vi "LinearSystemLoop_DCMotor_Execute.vi"(5 "LinearSystem_ID_DCMotor_Model":T2={"DCMOTOR_TYPES"=enum."NEO", "Num Motors"=1, "Gearing"=1.0, "MOI kgm2"=0.001} {"MOI kgm2" format="%#_13g"; "Gearing" format="%#_13g"}, 6 "dT Sec":dbl=0.02, 7 "LinearSystem_DCMotor_Ctrl_Params":T1={"Vel Model Std Dev Rad/Sec"=0.8, "Vel Meas Std Dev Rad/Sec"=0.02, "Vel Ctrl Tol Rad/Sec"=0.8, "Max Ctrl Out V"=12.0, "Pos Model Std Dev Rad"=0.8, "Pos Meas Std Dev Rad"=0.02, "Pos Ctrl Tol Rad"=0.8}, 8 "Position PV (Rad)":dbl format="%#_13g", 9 "Velocity (Rad/Sec)\n(PV)":dbl, 10 "Position SP (Rad)":dbl format="%#_13g", 11 "Velocity (Rad/Sec)\nSetpoint (SP)":dbl) -> (0 "Error":bool, 1 "Kalman Filtered Position (PV) Rad":dbl, 2 "Kalman FIltered\nVelocity (PV)":dbl, 3 "Motor Dmd":dbl, 4 "out Linear System Loop":T4)   [LabVIEW 2019, in "Trajectory_Library.lvlib"]
doc: "Model and control a DC Motor system using a Kalman FIlter and LQR controller. This is a single call LabVIEW function.\n\nThe DC Motor linear system is defined as:\n - states: \n - angular position (rad)\n - angular velocity (rad/sec)\n - inputs:\n - motor voltage\n - outputs: \n - angular position (rad) \n - angular velocity (rad/sec)\n\nInputs:\n - LinearSystemId DC Motor Model -- cluster -- Packed parameters used to create DC Motor linear system.\n - LineaarSystem DC Motor Ctrl -- cluster -- Packed parameters used by Kalman Filter and LQR to control the system.\n - Velocity Setpoint -- double -- Desired velocity (Rad/Sec)\n - Position Setpiont -- double -- Desired position (Radians, Default: 0)\n - Velocity -- double -- Measured velocity (Rad/Sec)\n - Position -- double -- Measured position (Radians)\n - dT -- double -- Update time (Seconds, Default: 0.02)\n\nOutputs:\n - Motor Dmd - double -- Motor demand (+/- 1.0)\n - Kalman FIltered Velocity -- double -- Filtered velocity (Rad/Sec)\n - Kalman FIltered Position -- double -- Filtered position (Radians)\n - Error -- boolean -- If TRUE an error occured."
uses:
  Trajectory_Library.lvlib
  TypeDef/LINEAR_SYSTEM_LOOP.ctl
  TypeDef/LINEAR_QUADRATIC_REGULATOR.ctl
  <vilib>/Analysis/Matrix/Datatypes/RealMatrix.ctl
  TypeDef/LINEAR_PLANT_INV_FF.ctl
  TypeDef/KALMAN_FILTER.ctl
  TypeDef/LINEAR_SYSTEM.ctl
  TypeDef/LINEAR_SYSTEM_ID_DCMOTOR_MODEL.ctl
  Enum/DCMOTOR_TYPES_ENUM.ctl
  TypeDef/LINEAR_SYSTEM_LOOP_DCMOTOR_CTRL_PARAMS.ctl
  MatBuilder_Create.vi
  DCMotor_GetCIM.vi
  DCMotor_GetAndymark9015.vi
  DCMotor_GetAndymarkRs775_125.vi
  DCMotor_GetBag.vi
  DCMotor_GetBanebotsRs550.vi
  DCMotor_GetBanebotsRs775.vi
  DCMotor_GetFalcon500.vi
  DCMotor_GetMiniCIM.vi
  DCMotor_GetNEO.vi
  DCMotor_GetNEO550.vi
  DCMotor_GetRomiBuiltIn.vi
  DCMotor_GetVex775Pro.vi
  DCMotor_GetAndymarkAM2235A.vi
  DCMotor_GetAndymarkAM3493.vi
  LinearSystem_New.vi
  MatrixHelper_Zero.vi
  MatBuilder_Fill.vi
  Matrix_Ident.vi
  DCMotor_New.vi
  Units_RotationsPerMinuteToRadiansPerSecond.vi
  MatrixHelper_CoerceSize.vi
  <vilib>/Analysis/7linalg.llb/Create Special Matrix.vi
  <vilib>/Analysis/7linalg.llb/Create Special Real Matrix.vi
  <vilib>/Analysis/Matrix/NI_Matrix.lvlib
panel:
  # "<States,1>"
  # "<FUTURE --- CLAMP TYPE -- For now\nuse Normalize>"
  # "Steady State Gain  \n<States,Outputs>"
  # "State Estimate <Statess,1>"
  # "<States,States>"
  # "<States,Inputs>"
  # "<Outputs,States>"
  # "<Outputs,Inputs>"
  # "<States,1>"
  # "<Inputs,1>"
  # "<States,Inputs>"
  # "<States,States>"
  # "Ref State <States,1>"
  # "Comp and capped \noutput <Inputs,1>"
  # "Controller gain\n<Inputs,States>"
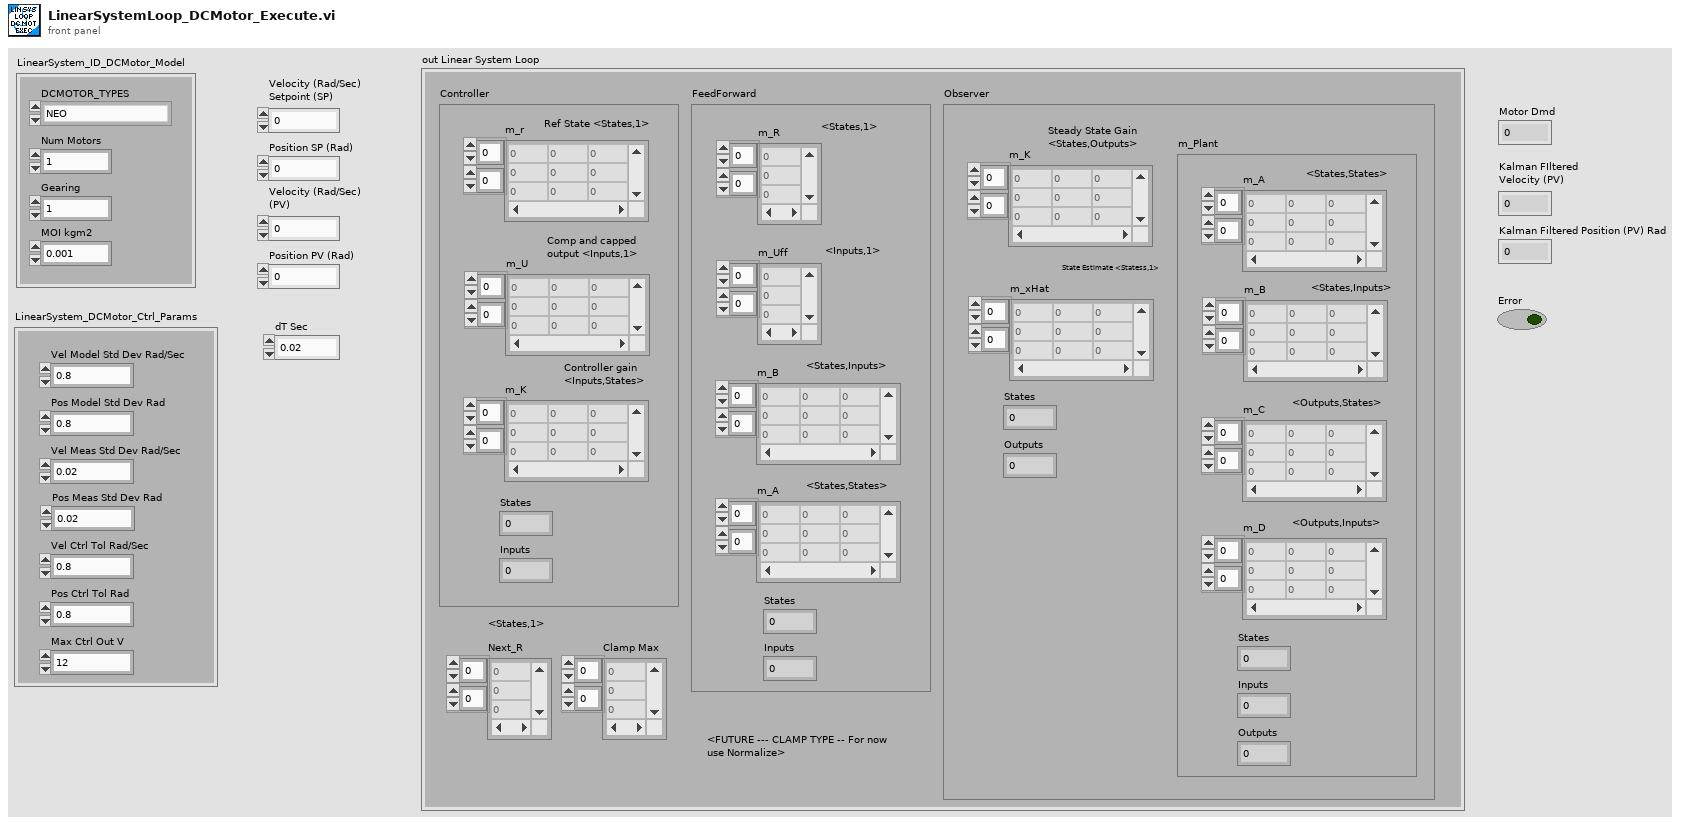
[diagram p1: front panel]
types:
  T1 = typedef "Trajectory_Library.lvlib/LINEAR_SYSTEM_LOOP_DCMOTOR_CTRL_PARAMS.ctl" = cluster{"Vel Model Std Dev Rad/Sec":dbl, "Vel Meas Std Dev Rad/Sec":dbl, "Vel Ctrl Tol Rad/Sec":dbl, "Max Ctrl Out V":dbl, "Pos Model Std Dev Rad":dbl, "Pos Meas Std Dev Rad":dbl, "Pos Ctrl Tol Rad":dbl}
  T2 = typedef "Trajectory_Library.lvlib/LINEAR_SYSTEM_ID_DCMOTOR_MODEL.ctl" = cluster{"DCMOTOR_TYPES":T3, "Num Motors":i32, "Gearing":dbl, "MOI kgm2":dbl}
  T3 = typedef "Trajectory_Library.lvlib/DCMOTOR_TYPES_ENUM.ctl" = enum16{"CIM", "AndyMark 9015", "Andy Mark RS 775 125", "Bag", "BaneBots RS 550", "BaneBots RS 775", "Falcon 500", "Mini CIM", "NEO", "NEO 550", "Romi BuiltIn", "Vex 775 Pro", "Snow Blower AM 2235A", "Bosch Seat AM 3493"}
  T4 = typedef "Trajectory_Library.lvlib/LINEAR_SYSTEM_LOOP.ctl" = cluster{"Controller":T5, "FeedForward":T7, "Observer":T8, "Next_R":T6, "Clamp Max":T6}
  T5 = typedef "Trajectory_Library.lvlib/LINEAR_QUADRATIC_REGULATOR.ctl" = cluster{"m_r":T6, "m_U":T6, "m_K":T6, "States":i32, "Inputs":i32}
  T6 = typedef "NI_Matrix.lvlib/RealMatrix.ctl" = dbl[][]
  T7 = typedef "Trajectory_Library.lvlib/LINEAR_PLANT_INV_FF.ctl" = cluster{"m_R":T6, "m_Uff":T6, "m_B":T6, "m_A":T6, "States":i32, "Inputs":i32}
  T8 = typedef "Trajectory_Library.lvlib/KALMAN_FILTER.ctl" = cluster{"m_K":T6, "m_xHat":T6, "States":i32, "Outputs":i32, "m_Plant":T9}
  T9 = typedef "Trajectory_Library.lvlib/LINEAR_SYSTEM.ctl" = cluster{"m_A":T6, "m_B":T6, "m_C":T6, "m_D":T6, "States":i32, "Inputs":i32, "Outputs":i32}
  T10 = typedef "Trajectory_Library.lvlib/DCMOTOR.CTL" = cluster{"nominalVoltage_Volts":dbl, "StallTorque_NM":dbl, "StallCurrent_Amps":dbl, "FreeCurrent_Amps":dbl, "FreeSpeed_RadPerSec":dbl, "R_Ohms":dbl, "KvINV_RadPerSecPerVolt":dbl, "Kt_NMPerAmp":dbl, "L_H":dbl, "Jr_KgM2":dbl}
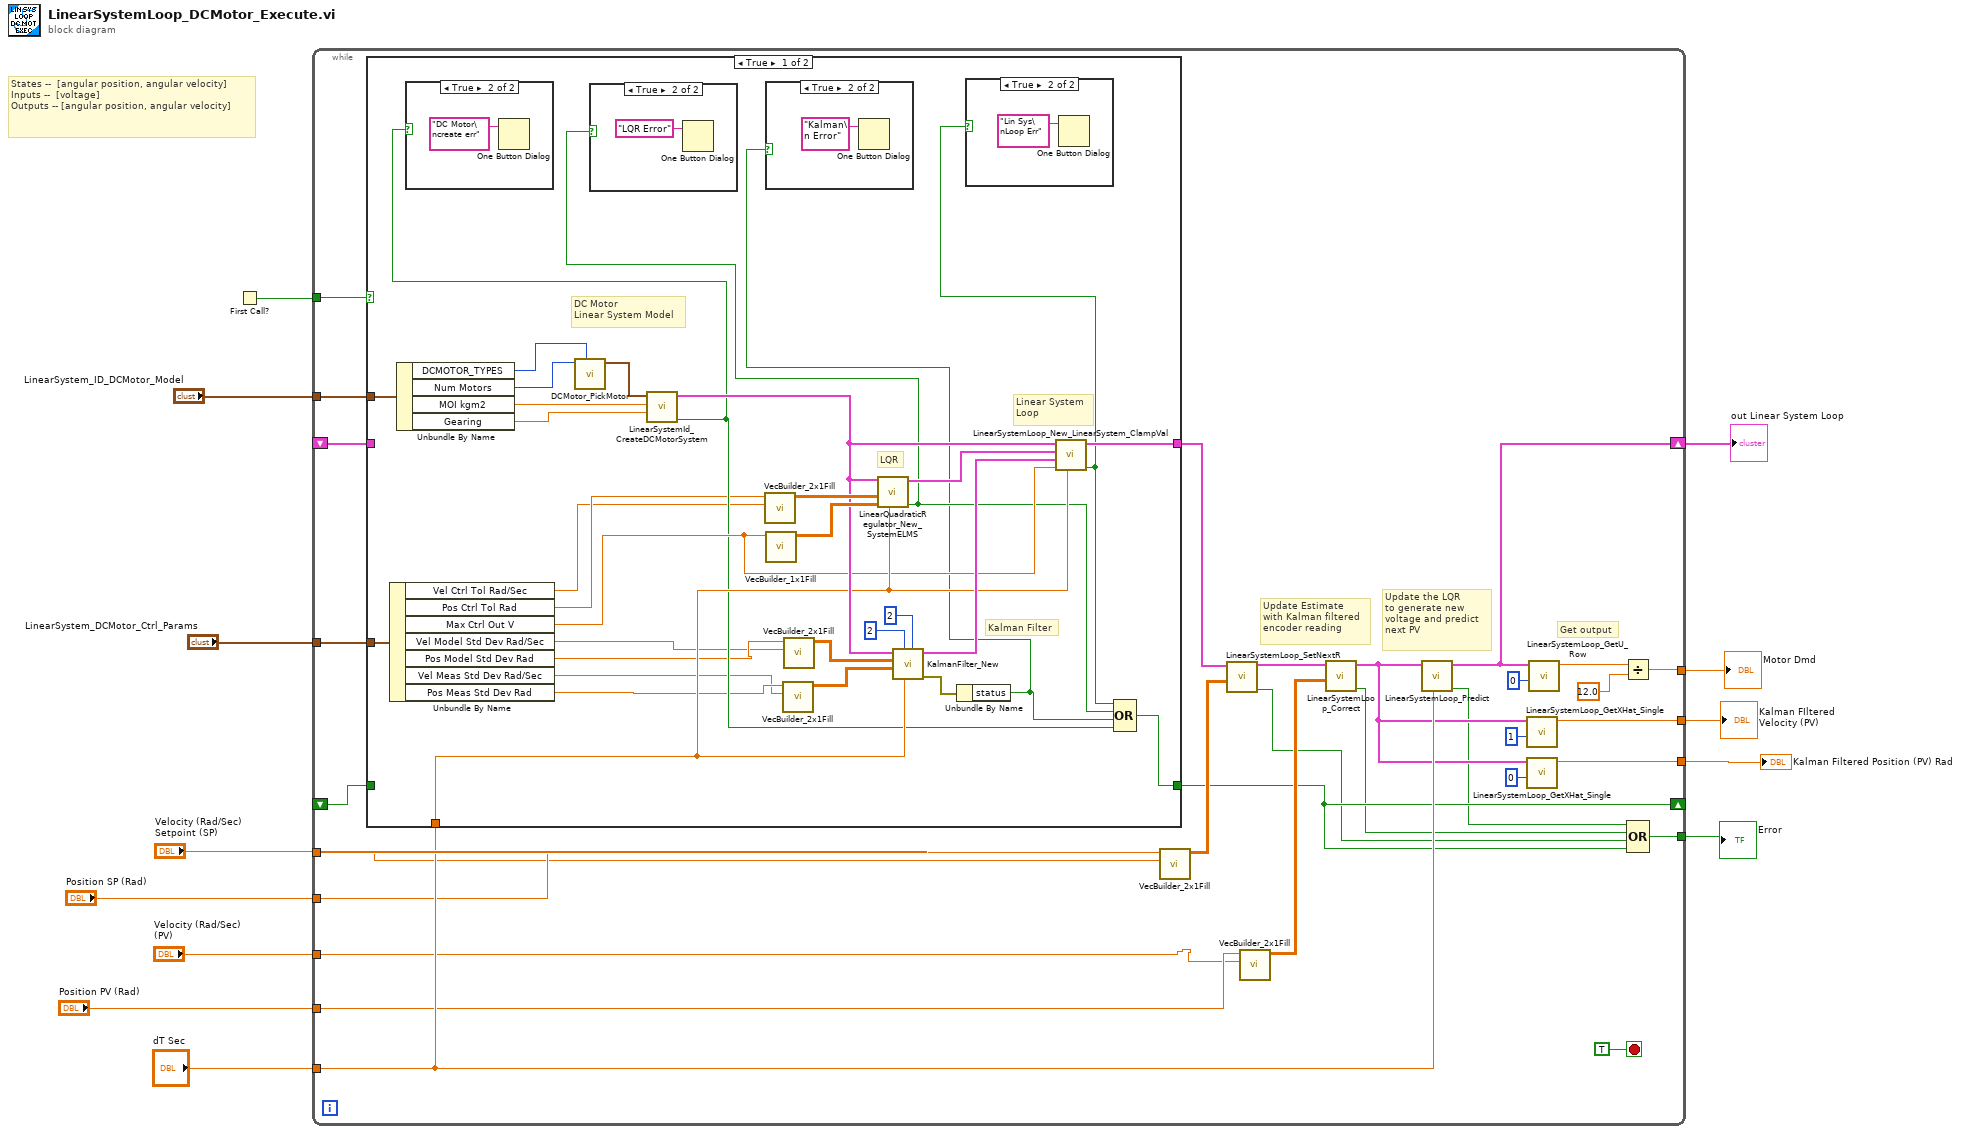
[diagram p0: block diagram]
diagram:
  # "States --  [angular position, angular velocity]\nInputs --  [voltage]\nOutputs -- [angular position, angular velocity]"
  n1 = First Call?() -> (First Call?: T/F=w8:bool)
  n2 = while {
    tunnel: "Velocity (Rad/Sec)\n(PV)" -> [w18]
    tunnel: [w29] -> w12
    tunnel: [w38] -> w11
    tunnel: "Position PV (Rad)" -> [w19]
    tunnel: "Velocity (Rad/Sec)\nSetpoint (SP)" -> [w20]
    tunnel: w8 -> [w35]
    tunnel: "LinearSystem_ID_DCMotor_Model" -> [w34]
    shift-right: [w22] -> w1
    shift-left: _ -> [w32]
    tunnel: "Position SP (Rad)" -> [w21]
    tunnel: "dT Sec" -> [w31]
    tunnel: "LinearSystem_DCMotor_Ctrl_Params" -> [w28]
    shift-right: [w17] -> _
    shift-left: _ -> [w27]
    tunnel: [w26] -> w3
    tunnel: [w23] -> w2
    stop <- TRUE stop-if-true
    # "Get output"
    # "Update the LQR \nto generate new \nvoltage and predict \nnext PV"
    # "Update Estimate\nwith Kalman filtered\nencoder reading"
    n3 = case shown="True" w35 {
      tunnel: w34 -> [w73 _]
      tunnel: [w59 w80] -> w33
      tunnel: w32 -> [_ w80]
      tunnel: w31 -> [w58 _]
      tunnel: w28 -> [w57 _]
      tunnel: [w55 w79] -> w17
      tunnel: w27 -> [_ w79]
      frame True {
        # "LQR"
        # "Linear System \nLoop"
        # "Kalman Filter"
        # "DC Motor\nLinear System Model"
        n4 = Unbundle By Name(w57) -> ("Vel Ctrl Tol Rad/Sec"=w50:dbl, "Pos Ctrl Tol Rad"=w51:dbl, "Max Ctrl Out V"=w56:dbl, "Vel Model Std Dev Rad/Sec"=w48:dbl, "Pos Model Std Dev Rad"=w49:dbl, "Vel Meas Std Dev Rad/Sec"=w46:dbl, "Pos Meas Std Dev Rad"=w47:dbl)
        n5 = Unbundle By Name(w73) -> ("DCMOTOR_TYPES"=w72:T3, "Num Motors"=w71:i32, "MOI kgm2"=w70:dbl, "Gearing"=w69:dbl)
        n6 = call "DCMotor_PickMotor.vi"("DCMOTOR_TYPES"=w72, "Num Motors"=w71) -> ("DCMOTOR"=w74:T10)  [unwired: 9 in]
        n7 = call "LinearSystemId_CreateDCMotorSystem.vi"("G"=w69, "jKgMetersSquared"=w70, "DCMOTOR"=w74) -> ("Error"=w54:bool, "Linearsystem"=w60:T9)  [unwired: 7 in]
        n8 = case shown="True" w54 {
          frame False {
          }
          frame True {
            n9 = One Button Dialog(message="DC Motor\ncreate err") -> ()  [unwired: 1 in, 1 out]
          }
        }
        n10 = call "VecBuilder_2x1Fill.vi"("R1"=w50, "R0"=w51) -> ("output matrix"=w61:T6)  [unwired: 9 in]
        n11 = call "VecBuilder_1x1Fill.vi"("R0_C0"=w56) -> ("output matrix"=w62:T6)  [unwired: 10 in]
        n12 = call "VecBuilder_2x1Fill.vi"("R1"=w46, "R0"=w47) -> ("output matrix"=w66:T6)  [unwired: 9 in]
        n13 = call "VecBuilder_2x1Fill.vi"("R1"=w48, "R0"=w49) -> ("output matrix"=w65:T6)  [unwired: 9 in]
        n14 = call "LinearQuadraticRegulator_New_SystemELMS.vi"("dt_Seconds"=w58, "Relms"=w62, "Qelms"=w61, "LINEARSYSTEM"=w60) -> ("Error"=w53:bool, "LinearQuadraticRegulator"=w67:T5)  [unwired: 6 in]
        n15 = case shown="True" w53 {
          frame False {
          }
          frame True {
            n16 = One Button Dialog(message="LQR Error") -> ()  [unwired: 1 in, 1 out]
          }
        }
        n17 = call "KalmanFilter_New.vi"("States"=2, "dt_Seconds"=w58, "Outputs"=2, "MeasurementStdDevs"=w66, "StateStdDevs"=w65, "Plant"=w60) -> ("Error"=w45:errorcluster, "KalmanFilter"=w68:T8)  [unwired: 4 in]
        n18 = Unbundle By Name(w45) -> ("status"=w44:bool)
        n19 = case shown="True" w44 {
          frame False {
          }
          frame True {
            n20 = One Button Dialog(message="Kalman\n Error") -> ()  [unwired: 1 in, 1 out]
          }
        }
        n21 = call "LinearSystemLoop_New_LinearSystem_ClampVal.vi"("dT_Seconds"=w58, "Max_Voltage"=w56, "Observer"=w68, "Controller"=w67, "Plant"=w60) -> ("Error"=w52:bool, "Linear System Loop"=w59:T4)  [unwired: 5 in]
        n22 = case shown="True" w52 {
          frame False {
          }
          frame True {
            n23 = One Button Dialog(message="Lin Sys\nLoop Err") -> ()  [unwired: 1 in, 1 out]
          }
        }
        n24 = Compound Arithmetic op=OR(w52, w53, w44, w54) -> (w55:bool)
      }
      frame False {
      }
    }
    n25 = call "VecBuilder_2x1Fill.vi"("R1"=w20, "R0"=w21) -> ("output matrix"=w37:T6)  [unwired: 9 in]
    n26 = call "LinearSystemLoop_SetNextR.vi"("R"=w37, "input inear System Loop"=w33) -> ("Size Coerced"=w16:bool, "out Linear System Loop"=w41:T4)  [unwired: 8 in]
    n27 = call "VecBuilder_2x1Fill.vi"("R1"=w18, "R0"=w19) -> ("output matrix"=w42:T6)  [unwired: 9 in]
    n28 = call "LinearSystemLoop_Correct.vi"("Y"=w42, "input inear System Loop"=w41) -> ("Error"=w15:bool, "out Linear System Loop"=w24:T4)  [unwired: 8 in]
    n29 = call "LinearSystemLoop_Predict.vi"("dT_Seconds"=w31, "input inear System Loop"=w24) -> ("Error"=w14:bool, "out Linear System Loop"=w22:T4)  [unwired: 8 in]
    n30 = call "LinearSystemLoop_GetXHat_Single.vi"("Row"=1, "input inear System Loop"=w24) -> ("XHat"=w29:dbl)  [unwired: 9 in]
    n31 = call "LinearSystemLoop_GetXHat_Single.vi"("Row"=0, "input inear System Loop"=w24) -> ("XHat"=w23:dbl)  [unwired: 9 in]
    n32 = call "LinearSystemLoop_GetU_Row.vi"("Row"=0, "input inear System Loop"=w22) -> ("U"=w39:dbl)  [unwired: 9 in]
    n33 = Divide(x=w39, y=12.0) -> (x/y=w38:dbl)
    n34 = Compound Arithmetic op=OR(w14, w15, w16, w17) -> (w26:bool)
  }
  "Motor Dmd" <- w11
  "out Linear System Loop" <- w1
  "Error" <- w3
  "Kalman FIltered\nVelocity (PV)" <- w12
  "Kalman Filtered Position (PV) Rad" <- w2
